vi "test Set AccessType.vi"(11 "Test Case In":refnum<class "test Electronic Datasheet.lvclass">) -> (0 "error out":errorcluster, 3 "Test Case Out":refnum<class "test Electronic Datasheet.lvclass">)   [LabVIEW 2024, in "test Electronic Datasheet.lvclass"]
uses:
  test Electronic Datasheet.lvclass
  C:/Program Files/National Instruments/LabVIEW 2024/vi.lib/Astemes/LUnit/Test Case.lvclass
  <vilib>/Astemes/LUnit/Test Case.lvclass/Test Case.ctl
  <vilib>/Astemes/LUnit/Append Pass Result.vi
  <vilib>/Astemes/LUnit/Append Fail Result.vi
  <vilib>/Astemes/LUnit/Run In UI.vi
  <vilib>/Utility/error.llb/Clear Errors.vi
  <vilib>/Astemes/LUnit/Test Case.lvclass
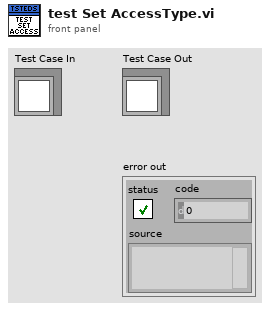
[diagram p1: front panel]
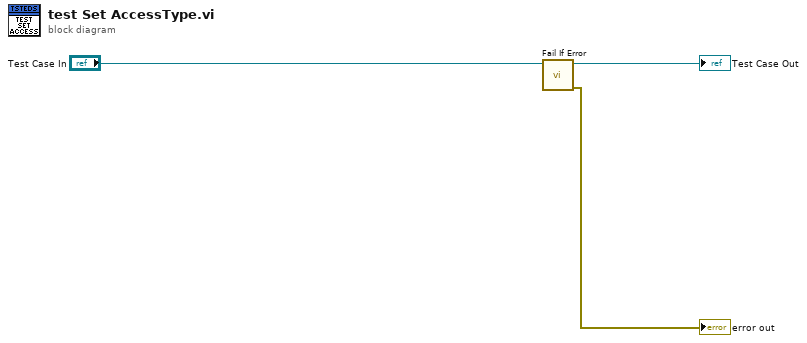
[diagram p0: block diagram]
diagram:
  n1 = call <vilib>:"Fail If Error.vi"("LUnit Test Case In"="Test Case In") -> ("error out"=→"error out":errorcluster, "LUnit Test Case Out"=→"Test Case Out":refnum<class "test Electronic Datasheet.lvclass">)  [unwired: 9 in]
